vi "Encoder_Read.vi"(7 "Reset Counter":bool, 8 "error in (no error)":errorcluster, 10 "B/BL Motor":T1 items=["BLDC", "BDC"], 11 "PORT":T2) -> (0 "error out":errorcluster, 2 "Rotations":dbl, 3 "RPM":dbl)   [LabVIEW 2019, in "Motor_Lib.lvlib"]
uses:
  Motor_Lib.lvlib
  PORT_ID.ctl
  MotorType.ctl
  <vilib>/myRIO/Instrument Drivers/Onboard IO/Encoder/typedefs/Encoder Reference.ctl
  <vilib>/myRIO/Common/Instrument Driver Framework/Utilities/typedefs/myRIO Generic Hardware Reference.ctl
  <vilib>/myRIO/Common/Instrument Driver Framework/Utilities/typedefs/Hardware Version Enum.ctl
  <vilib>/myRIO/Common/Instrument Driver Framework/Utilities/typedefs/myRIO v1.0 Reference.ctl
  <vilib>/myRIO/Common/Instrument Driver Framework/Utilities/typedefs/Generic FPGA Reference.ctl
  <vilib>/myRIO/Common/Instrument Driver Framework/myRIO v1.0/Encoder/typedefs/Encoder Channels Enum.ctl
  <vilib>/myRIO/Common/Instrument Driver Framework/myRIO v1.0/Encoder/typedefs/Encoder Signal Mode.ctl
  <vilib>/userDefined/High Color/nirio_resource_hc.ctl
  <vilib>/myRIO/Common/Instrument Driver Framework/myRIO v1.0/Encoder/typedefs/Encoder Configuration v1.0.ctl
  <vilib>/myRIO/Instrument Drivers/Onboard IO/Encoder/vis/Read.vi
  <vilib>/myRIO/Common/Instrument Driver Framework/myRIO v1.0/Encoder/vis/myRIO v1.1 Open Encoder.vi
  <vilib>/myRIO/Common/Instrument Driver Framework/Utilities/vis/Is FPGA Ref Available.vi
  <vilib>/myRIO/Common/Instrument Driver Framework/Utilities/vis/Validate Channels.vi
  <vilib>/myRIO/Common/Instrument Driver Framework/myRIO v1.0/Encoder/vis/myRIO v1.0 Reserve Encoder.vi
  <vilib>/myRIO/Common/Instrument Driver Framework/myRIO v1.0/Encoder/vis/myRIO v1.0 Build MUX Configuration Encoder.vi
  <vilib>/myRIO/Common/Instrument Driver Framework/myRIO v1.0/Resource Manager/vis/myRIO v1.0 Reserve Channel List.vi
  <vilib>/myRIO/Common/Instrument Driver Framework/myRIO v1.0/Resource Manager/vis/myRIO v1.0 Create Configuration List.vi
  <vilib>/myRIO/Common/Instrument Driver Framework/myRIO v1.0/Resource Manager/vis/myRIO v1.0 Reserve Channel.vi
  <vilib>/myRIO/Common/Instrument Driver Framework/myRIO v1.0/Resource Manager/vis/myRIO v1.0 Unreserve Channel.vi
  <vilib>/myRIO/Common/Instrument Driver Framework/myRIO v1.0/Resource Manager/vis/myRIO v1.0 Build Mutex Name.vi
  <vilib>/Utility/VariantDataType/GetNumericInfo.vi
  <vilib>/Utility/error.llb/Error Cluster From Error Code.vi
  <vilib>/myRIO/Common/Instrument Driver Framework/myRIO v1.0/myRIO v1.1 Open.vi
  <vilib>/myRIO/Common/Instrument Driver Framework/Utilities/vis/IO Manager.vi
  <vilib>/myRIO/Common/Instrument Driver Framework/Utilities/vis/Configuration Manager.vi
  <vilib>/myRIO/Common/Instrument Driver Framework/myRIO v1.0/Resource Manager/vis/myRIO v1.0 Configure IO.vi
  <vilib>/myRIO/Common/Instrument Driver Framework/myRIO v1.0/myRIO v1.0 Close.vi
  <vilib>/myRIO/Common/Instrument Driver Framework/myRIO v1.0/Encoder/vis/myRIO v1.0 Configure Encoder.vi
  <vilib>/myRIO/Common/Instrument Driver Framework/myRIO v1.0/Encoder/vis/myRIO v1.0 Read Encoder.vi
  <vilib>/myRIO/Express VI/Onboard IO/Encoder/Encoder Express VI.xnode
  <vilib>/myRIO/Instrument Drivers/Onboard IO/Encoder/vis/myRIO Encoder Open.xnode
  <vilib>/myRIO/Common/Instrument Driver Framework/myRIO v1.0/Encoder/typedefs/Encoder Count Direction Enum.ctl
  <vilib>/myRIO/Instrument Drivers/Onboard IO/Encoder/Encoder.lvlib
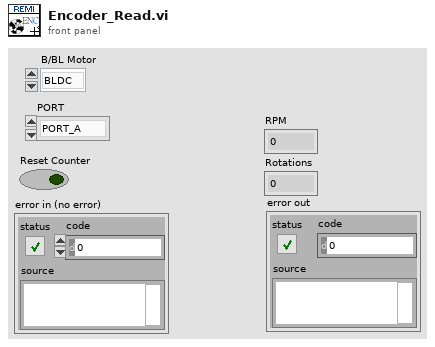
[diagram p1: front panel]
types:
  T1 = typedef "Motor_Lib.lvlib/MotorType.ctl" = u16
  T2 = typedef "Motor_Lib.lvlib/PORT_ID.ctl" = enum16{"PORT_A", "PORT_B"}
  T3 = typedef "Encoder.lvlib/Encoder Reference.ctl" = cluster{"myRIO Reference":T4, "Encoder Channels Enum":T8}
  T4 = typedef "myRIO Generic Hardware Reference.ctl" = cluster{"myRIO Model":T5, "myRIO Hardware Reference":T6}
  T5 = typedef "Hardware Version Enum.ctl" = enum16{"Unknown", "myRIO-1900", "myRIO-1950", "roboRIO", "NI ELVIS RIO CM", "ELVIS III"}
  T6 = typedef "myRIO v1.0 Reference.ctl" = cluster{"Generic FPGA Reference":T7, "Allow multiple opens":bool}
  T7 = typedef "Generic FPGA Reference.ctl" = refnum<k20>
  T8 = typedef "Encoder Channels Enum.ctl" = enum16{"Not Connected", "C/ENC0", "C/ENC1", "A/ENC", "A/ENC0", "A/ENC1", "A/ENC2", "A/ENC3", "A/ENC4", "A/ENC5", "A/ENC6", "A/ENC7", "A/ENC8", "A/ENC9", "B/ENC", "B/ENC0", "B/ENC1", "B/ENC2", "B/ENC3", "B/ENC4", "B/ENC5", "B/ENC6", "B/ENC7", "B/ENC8", "B/ENC9", "DIO/ENC0", "DIO/ENC1", "DIO/ENC2", "DIO/ENC3", "DIO/ENC4"}
  T9 = typedef "Encoder Signal Mode.ctl" = enum16{"Quadrature phase signal", "Step and direction signal"}
  T10 = typedef "nirio_resource_hc.ctl" = tag
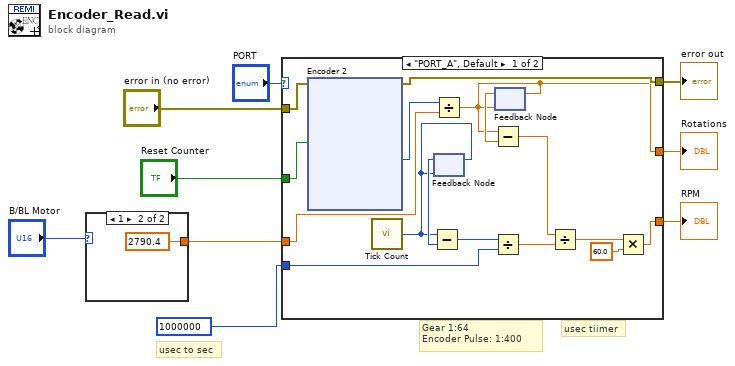
[diagram p0: block diagram]
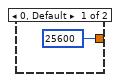
[diagram p2: hidden frame]
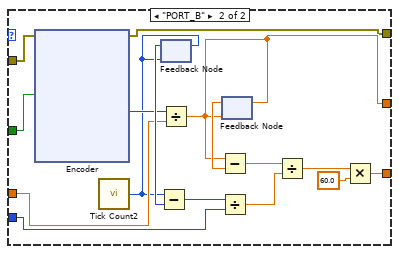
[diagram p3: hidden frame]
diagram:
  # "usec tiimer"
  # "usec to sec"
  # "Gear 1:64\nEncoder Pulse: 1:400"
  n1 = case shown="1" "B/BL Motor" {
    tunnel: [25600 ("y") 2790.4 ("y")] -> w1
    frame 0, Default {
    }
    frame 1 {
    }
  }
  n2 = case shown="\"PORT_A\", Default" "PORT" {
    tunnel: "Reset Counter" -> [w18 w89]
    tunnel: [w16 w80] -> w7
    tunnel: [w15 w79] -> w6
    tunnel: "error in (no error)" -> [w19 w78]
    tunnel: [w17 w77] -> w4
    tunnel: u32 1000000 ("y") -> [w13 w76]
    tunnel: w1 -> [w14 w75]
    frame "PORT_A", Default {
      n3 = xnode "Encoder 2"("Reset Counter"=w18, "error in (no error)"=w19) -> ("Counter Value"=w25:i32, "error out"=w17:errorcluster)  [unwired: 2 out]
      n4 = call "Tick Count"() -> ("Tick Count(uSec)"=w12:u32)
      n5 = Divide(x=w25, y=w14) -> (x/y=w15:dbl)
      n6 = feedback #1(w12) -> (w22:u32)
      n7 = Subtract(x=w12, y=w22) -> (x-y=w23:u32)
      n8 = feedback-in #1(w12) -> ()
      n9 = Divide(x=w23, y=w13) -> (x/y=w24:dbl)
      n10 = feedback #2(w15) -> (w21:dbl)
      n11 = Subtract(x=w15, y=w21) -> (x-y=w26:dbl)
      n12 = feedback-in #2(w15) -> ()
      n13 = Divide(x=w26, y=w24) -> (x/y=w27:dbl)
      n14 = Multiply(x=w27, y=60.0) -> (x*y=w16:dbl)
    }
    frame "PORT_B" {
      n15 = xnode "Encoder"("Reset Counter"=w89, "error in (no error)"=w78) -> ("Counter Value"=w84:i32, "error out"=w77:errorcluster)  [unwired: 2 out]
      n16 = call "Tick Count2"() -> ("Tick Count(uSec)"=w74:u32)
      n17 = feedback-in #3(w74) -> ()
      n18 = feedback #3(w74) -> (w87:u32)
      n19 = Subtract(x=w74, y=w87) -> (x-y=w86:u32)
      n20 = Divide(x=w84, y=w75) -> (x/y=w79:dbl)
      n21 = Divide(x=w86, y=w76) -> (x/y=w85:dbl)
      n22 = feedback #4(w79) -> (w88:dbl)
      n23 = Subtract(x=w79, y=w88) -> (x-y=w83:dbl)
      n24 = feedback-in #4(w79) -> ()
      n25 = Divide(x=w83, y=w85) -> (x/y=w82:dbl)
      n26 = Multiply(x=w82, y=60.0) -> (x*y=w80:dbl)
    }
  }
  "RPM" <- w7
  "Rotations" <- w6
  "error out" <- w4
